vi "KE622x -- Execute Diff Cond Meas.vi"(0 "Resource In":refnum<visa-resource-name>, 1 "Check For SCPI Errors? (T)":bool=TRUE, 5 "2812 -A Params In":T11={"Auto Range?"=FALSE, "Man / Selected\nRange"=enum."10mV", "Enable Digital\nFilter?"=FALSE, "Filter Type"=enum."Moving", "Filter Count"=10, "Filter\nWindow (%)"=0.01, "Enable Analog\nFilter?"=FALSE, "NPLCs"=5} {"Filter\nWindow (%)" min=0.0 max=10.0 step=0.01 format="%.2f"; "Filter Count" min=1 max=100; "NPLCs" min=1 max=10}, 7 "Differential Cond Params In":T3={"Start Value (A)"=-1e-05, "Stop Value (A)"=1e-05, "Step Size (A)"=1e-06, "Delta Value (A)"=1e-06, "Delay (s)"=0.001, "Abort On\nCompliance?"=FALSE} {"Delay (s)" min=0.001 max=9999.999 format="%.3f"; "Delta Value (A)" min=0.0 max=0.105 format="%.3p"; "Step Size (A)" min=0.0 max=0.105 format="%.3p"; "Stop Value (A)" min=-0.105 max=0.105 format="%.3p"; "Start Value (A)" min=-0.105 max=0.105 format="%.3p"}, 9 "Meas Units":T1, 11 "error in (no error)":errorcluster, 13 "Timeout (20000 ms)":u32=20000) -> (4 "Resource Out (dupl)":refnum<visa-resource-name>, 6 "2812 -A Params Out":T11={"Auto Range?"=FALSE, "Man / Selected\nRange"=enum."10mV", "Enable Digital\nFilter?"=FALSE, "Filter Type"=enum."Moving", "Filter Count"=10, "Filter\nWindow (%)"=0.01, "Enable Analog\nFilter?"=FALSE, "NPLCs"=5} {"Filter\nWindow (%)" min=0.0 max=10.0 step=0.01 format="%.2f"; "Filter Count" min=1 max=100; "NPLCs" min=1 max=60}, 8 "Differential Cond Params Out":T3={"Start Value (A)"=0.0, "Stop Value (A)"=-1e-05, "Step Size (A)"=1e-05, "Delta Value (A)"=1e-06, "Delay (s)"=1e-06, "Abort On\nCompliance?"=FALSE} {"Delay (s)" min=0.001 max=9999.999 format="%.3f"; "Delta Value (A)" min=0.0 max=0.105 format="%.3p"; "Step Size (A)" min=0.0 max=0.105 format="%.3p"; "Stop Value (A)" min=-0.105 max=0.105 format="%.3p"; "Start Value (A)" min=-0.105 max=0.105 format="%.3p"}, 10 "Timeout?":bool, 14 "Execution Time":dbl, 15 "error out":errorcluster)   [LabVIEW 2019, in "Keithley 622x.lvlib"]
doc: "Used to set up and execute a Differential Conductance Mode measurement. This VI accepts setup parameters for both the 2182/2182A and the 622x instruments."
uses:
  Keithley 622x.lvlib
  Configure/2182 -A/Low Level/Typedefs/KE2182 -- Voltage Ranges.ctl
  Configure/2182 -A/Low Level/Typedefs/KE2182 -- Filter Type.ctl
  Configure/2182 -A/Low Level/Typedefs/KE2182 -- Filter Count.ctl
  Configure/2182 -A/Low Level/Typedefs/KE2182 -- Filter Window.ctl
  Configure/2182 -A/Low Level/Typedefs/KE2182 -- NPLCs.ctl
  Configure/Delta PDelta DCon Modes/Typedefs/KE622x -- DCon Mode Params.ctl
  Configure/Delta PDelta DCon Modes/Low Level/Typedefs/KE622x -- DCon Mode Start Stop Level.ctl
  Configure/Delta PDelta DCon Modes/Low Level/Typedefs/KE622x -- DCon Mode Step Delta Size.ctl
  Configure/Delta PDelta DCon Modes/Low Level/Typedefs/KE622x -- Delta DCon Mode Delay.ctl
  Configure/Units/Typedefs/KE622x -- Voltage Meas Units.ctl
panel:
  out "Last Point Source Value (A)":T2=-1e-05 min=-0.105 max=0.105 format="%.3p"
  out "Num Points":u32
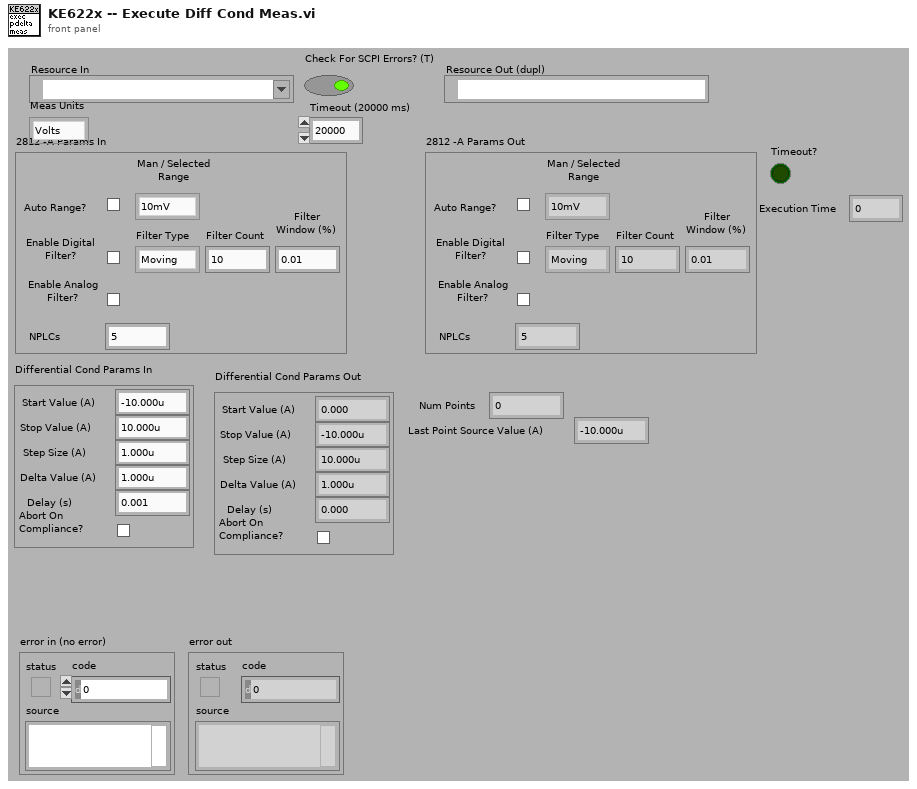
[diagram p1: front panel]
types:
  T1 = typedef "Keithley 622x.lvlib/KE622x -- Voltage Meas Units.ctl" = enum16{"Volts", "Ohms", "Watts", "Siemens"}
  T2 = typedef "Keithley 622x.lvlib/KE622x -- DCon Mode Start Stop Level.ctl" = dbl
  T3 = typedef "Keithley 622x.lvlib/KE622x -- DCon Mode Params.ctl" = cluster{"Start Value (A)":T2, "Stop Value (A)":T2, "Step Size (A)":T4, "Delta Value (A)":T4, "Delay (s)":T5, "Abort On\nCompliance?":bool}
  T4 = typedef "Keithley 622x.lvlib/KE622x -- DCon Mode Step Delta Size.ctl" = dbl
  T5 = typedef "Keithley 622x.lvlib/KE622x -- Delta DCon Mode Delay.ctl" = dbl
  T6 = typedef "Keithley 622x.lvlib/KE2182 -- Voltage Ranges.ctl" = enum16{"10mV", "100mV", "1V", "10V", "100V"}
  T7 = typedef "Keithley 622x.lvlib/KE2182 -- Filter Type.ctl" = enum16{"Moving", "Repeat"}
  T8 = typedef "Keithley 622x.lvlib/KE2182 -- Filter Count.ctl" = u32
  T9 = typedef "Keithley 622x.lvlib/KE2182 -- Filter Window.ctl" = dbl
  T10 = typedef "Keithley 622x.lvlib/KE2182 -- NPLCs.ctl" = u32
  T11 = cluster{"Auto Range?":bool, "Man / Selected\nRange":T6, "Enable Digital\nFilter?":bool, "Filter Type":T7, "Filter Count":T8, "Filter\nWindow (%)":T9, "Enable Analog\nFilter?":bool, "NPLCs":T10}
  T12 = typedef "Keithley 622x.lvlib/KE622x -- Meas Event Reg State.ctl" = cluster{"B0, ROF:  KE2182A Delta Reading Overflow Event?":bool, "B1, Int:  Interlock OK Event?":bool, "B2, Temp:  Over Temperature Event?":bool, "B3, Comp:  Compliance Event?":bool, "B5, RAV:  Delta Reading Available Event?":bool, "B6, TN:  User Defined Reading Number Stored In Buffer Event?":bool, "B7, BAV:  At Least 2 Readings Stored In Buffer Event?":bool, "B12, BQF:  Buffer Quarter Full Event?":bool, "B8, BHF:  Buffer Half Full Event?":bool, "B13, B3QF:  Buffer 3/4 Full Event?":bool, "B9, BFL:  Buffer Full Event?":bool}
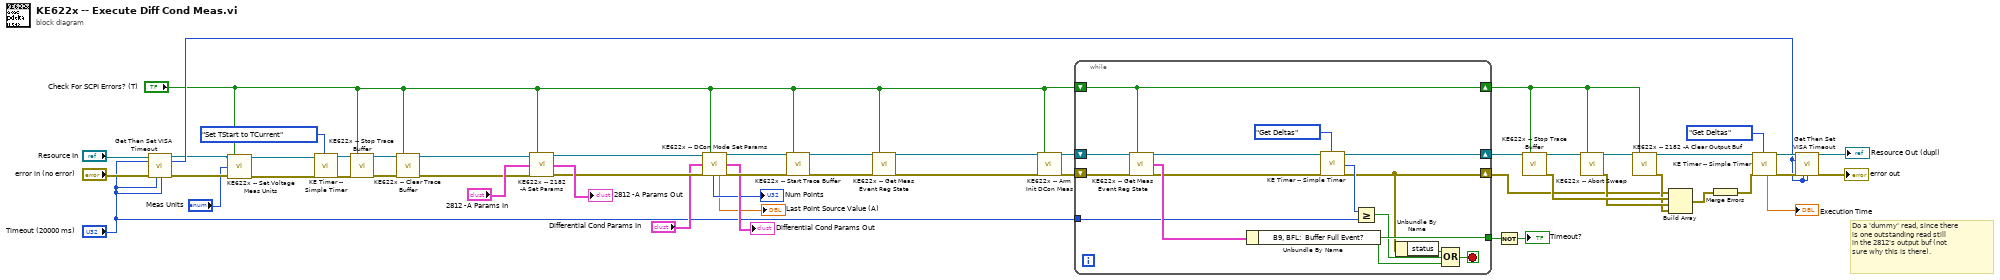
[diagram p0: block diagram]
diagram:
  # "Do a 'dummy' read, since there\nis one outstanding read still\nin the 2812's output buf (not\nsure why this is there)."
  n1 = call "Get Then Set VISA Timeout.vi"("VISA Resource Name In"="Resource In", "New Timeout (msecs)"="Timeout (20000 ms)", "error in (no error)"="error in (no error)", "Max Timeout (300 secs)"="Timeout (20000 ms)", "Min Timeout (3 secs)"="Timeout (20000 ms)") -> ("VISA Resource Name Out (dupl)"=w6:refnum<visa-resource-name>, "Old Timeout (msecs)"=w9:u32, "error out"=w5:errorcluster)  [unwired: 7 in, 1 out]
  n2 = call "KE622x -- Set Voltage Meas Units.vi"("Resource In"=w6, "Check For SCPI Errors? (T)"="Check For SCPI Errors? (T)", "Voltage Meas Units"="Meas Units", "error in (no error)"=w5) -> ("Resource Out (dupl)"=w3:refnum<visa-resource-name>, "error out"=w2:errorcluster)  [unwired: 10 in]
  n3 = call "KE Timer -- Simple Timer.vi"("Resource In"=w3, "error in (no error)"=w2, "Action"=enum16{"Set TStart to TCurrent", "Get Deltas"}."Set TStart to TCurrent") -> ("Resource Out (dupl)"=w30:refnum<visa-resource-name>, "error out (dupl)"=w29:errorcluster)  [unwired: 7 in, 8 out]
  n4 = call "KE622x -- Stop Trace Buffer.vi"("Resource In"=w30, "Check For SCPI Errors? (T)"="Check For SCPI Errors? (T)", "error in (no error)"=w29) -> ("Resource Out (dupl)"=w48:refnum<visa-resource-name>, "error out"=w47:errorcluster)  [unwired: 11 in]
  n5 = call "KE622x -- Clear Trace Buffer.vi"("Resource In"=w48, "Check For SCPI Errors? (T)"="Check For SCPI Errors? (T)", "error in (no error)"=w47) -> ("Resource Out (dupl)"=w28:refnum<visa-resource-name>, "error out"=w27:errorcluster)  [unwired: 11 in]
  n6 = call "KE622x -- 2182 -A Set Params.vi"("622x Resource In"=w28, "Check For SCPI Errors? (T)"="Check For SCPI Errors? (T)", "2812 -A Params In"="2812 -A Params In", "error in (no error)"=w27) -> ("622x Resource Out (dupl)"=w50:refnum<visa-resource-name>, "2812 -A Params Out"=→"2812 -A Params Out":T11, "error out"=w49:errorcluster)  [unwired: 9 in]
  n7 = call "KE622x -- DCon Mode Set Params.vi"("Resource In"=w50, "Check For SCPI Errors? (T)"="Check For SCPI Errors? (T)", "Differential Cond Params In"="Differential Cond Params In", "error in (no error)"=w49) -> ("Resource Out (dupl)"=w46:refnum<visa-resource-name>, "Differential Cond Params Out"=→"Differential Cond Params Out":T3, "Num Buf Points"=→"Num Points":u32, "Last Buf Point Source Value (A)"=→"Last Point Source Value (A)":T2, "error out"=w45:errorcluster)  [unwired: 7 in]
  n8 = call "KE622x -- Start Trace Buffer.vi"("Resource In"=w46, "Check For SCPI Errors? (T)"="Check For SCPI Errors? (T)", "error in (no error)"=w45) -> ("Resource Out (dupl)"=w43:refnum<visa-resource-name>, "error out"=w44:errorcluster)  [unwired: 11 in]
  n9 = call "KE622x -- Get Meas Event Reg State.vi"("VISA Resource In"=w43, "Error Query (T)?"="Check For SCPI Errors? (T)", "error in (no error)"=w44) -> ("VISA Resource Out (dupl)"=w11:refnum<visa-resource-name>, "error out"=w10:errorcluster)  [unwired: 10 in, 1 out]
  n10 = call "KE622x -- Arm Init DCon Meas.vi"("Resource In"=w11, "Check For SCPI Errors? (T)"="Check For SCPI Errors? (T)", "error in (no error)"=w10) -> ("Resource Out (dupl)"=w40:refnum<visa-resource-name>, "error out"=w41:errorcluster)  [unwired: 11 in]
  n11 = while {
    shift-right: [w54] -> w17
    shift-left: w41 -> [w67]
    shift-right: [w57] -> w37
    shift-left: w40 -> [w66]
    tunnel: [w59] -> w39
    shift-right: [w56] -> w34
    shift-left: "Check For SCPI Errors? (T)" -> [w56]
    tunnel: "Timeout (20000 ms)" -> [w53]
    stop <- w60 stop-if-true
    n12 = call "KE622x -- Get Meas Event Reg State.vi"("VISA Resource In"=w66, "Error Query (T)?"=w56, "error in (no error)"=w67) -> ("VISA Resource Out (dupl)"=w63:refnum<visa-resource-name>, "KE622x Meas Event Reg"=w65:T12, "error out"=w64:errorcluster)  [unwired: 10 in]
    n13 = Unbundle By Name(w65) -> ("B9, BFL:  Buffer Full Event?"=w59:bool)
    n14 = call "KE Timer -- Simple Timer.vi"("Resource In"=w63, "error in (no error)"=w64, "Action"=enum16{"Set TStart to TCurrent", "Get Deltas"}."Get Deltas") -> ("Resource Out (dupl)"=w57:refnum<visa-resource-name>, "TCurrent - TStart (ms)"=w61:u32, "error out (dupl)"=w54:errorcluster)  [unwired: 7 in, 7 out]
    n15 = Greater Or Equal?(x=w61, y=w53) -> (x >= y?=w58:bool)
    n16 = Unbundle By Name(w54) -> ("status"=w55:bool)
    n17 = Compound Arithmetic op=OR(w55, w58, w59) -> (w60:bool)
  }
  n18 = Not(x=w39) -> (.not. x?=→"Timeout?":bool)
  n19 = call "KE622x -- Stop Trace Buffer.vi"("Resource In"=w37, "Check For SCPI Errors? (T)"=w34) -> ("Resource Out (dupl)"=w36:refnum<visa-resource-name>, "error out"=w26:errorcluster)  [unwired: 12 in]
  n20 = call "KE622x -- Abort Sweep.vi"("Resource In"=w36, "Check For SCPI Errors? (T)"=w34) -> ("Resource Out (dupl)"=w35:refnum<visa-resource-name>, "error out"=w25:errorcluster)  [unwired: 12 in]
  n21 = call "KE622x -- 2182 -A Clear Output Buf.vi"("622x Resource In"=w35, "Check For SCPI Errors? (T)"=w34) -> ("622x Resource Out (dupl)"=w33:refnum<visa-resource-name>, "error out"=w24:errorcluster)  [unwired: 11 in, 1 out]
  n22 = Build Array(w17, w26, w25, w24) -> (w23:errorcluster[])
  n23 = Merge Errors(w23) -> (w18:errorcluster)
  n24 = call "KE Timer -- Simple Timer.vi"("Resource In"=w33, "error in (no error)"=w18, "Action"=enum16{"Set TStart to TCurrent", "Get Deltas"}."Get Deltas") -> ("TCurrent - TStart (s)"=→"Execution Time":dbl, "Resource Out (dupl)"=w14:refnum<visa-resource-name>, "error out (dupl)"=w13:errorcluster)  [unwired: 7 in, 7 out]
  n25 = call "Get Then Set VISA Timeout.vi"("VISA Resource Name In"=w14, "New Timeout (msecs)"=w9, "error in (no error)"=w13, "Max Timeout (300 secs)"=w9, "Min Timeout (3 secs)"=w9) -> ("VISA Resource Name Out (dupl)"=→"Resource Out (dupl)":refnum<visa-resource-name>, "error out"=→"error out":errorcluster)  [unwired: 7 in, 2 out]
